vi "Ejercicio4_Aprobado-Reprobado.vi"() -> ()   [LabVIEW 2022 SP3]
panel:
  in  "stop":bool
  out "Reprobado":bool
  out "Aprobado":bool
  in  "Calificación":dbl
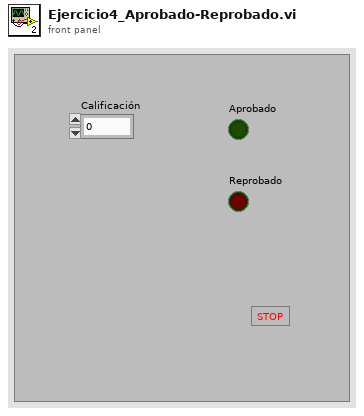
[diagram p1: front panel]
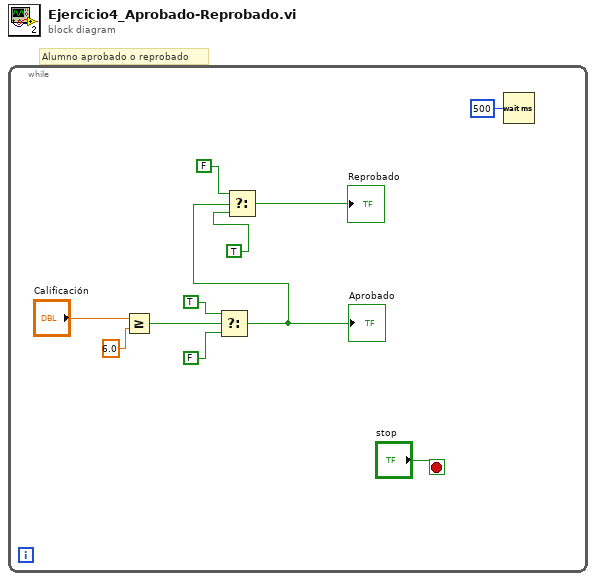
[diagram p0: block diagram]
diagram:
  # "Alumno aprobado o reprobado"
  n1 = while {
    stop <- "stop" stop-if-true
    n2 = Greater Or Equal?(x="Calificación", y=6.0) -> (x >= y?=w7:bool)
    n3 = Select(t=TRUE, s=w7, f=FALSE) -> (s? t:f=w2:bool)
    "Aprobado" <- w2
    n4 = Select(t=FALSE, s=w2, f=TRUE) -> (s? t:f=→"Reprobado":bool)
    n5 = Wait (ms)(milliseconds to wait=u32 500) -> ()  [unwired: 1 out]
  }
